vi "PS-RA01B FPGA.vi"() -> ()   [LabVIEW 2011]
uses:
  <vilib>/rvi/eio/common/nirviEmuTemplateMethod_errors.vi
  <vilib>/eio/EIONode/EIONode.xnode
  <vilib>/rvi/Analysis/measure/butterworth/XNode/niFpgaButterworthFilter.xnode
  <vilib>/eio/EIOMethodNode/EIOMethodNode.xnode
panel:
  out "Mod5/AI2":fxp<+/-,20,5> format="%.17g"
  out "Mod5/AI0":fxp<+/-,20,5> format="%.17g"
  out "Mod5/AI1":fxp<+/-,20,5> format="%.17g"
  out "Mod1/AI2":fxp<+/-,20,5> format="%.17g"
  out "Mod1/AI3":fxp<+/-,20,5> format="%.17g"
  out "Mod1/AI0":fxp<+/-,20,5> format="%.17g"
  out "Mod1/AI1":fxp<+/-,20,5> format="%.17g"
  out "Mod5/AI3":fxp<+/-,20,5> format="%.17g"
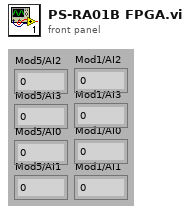
[diagram p1: front panel]
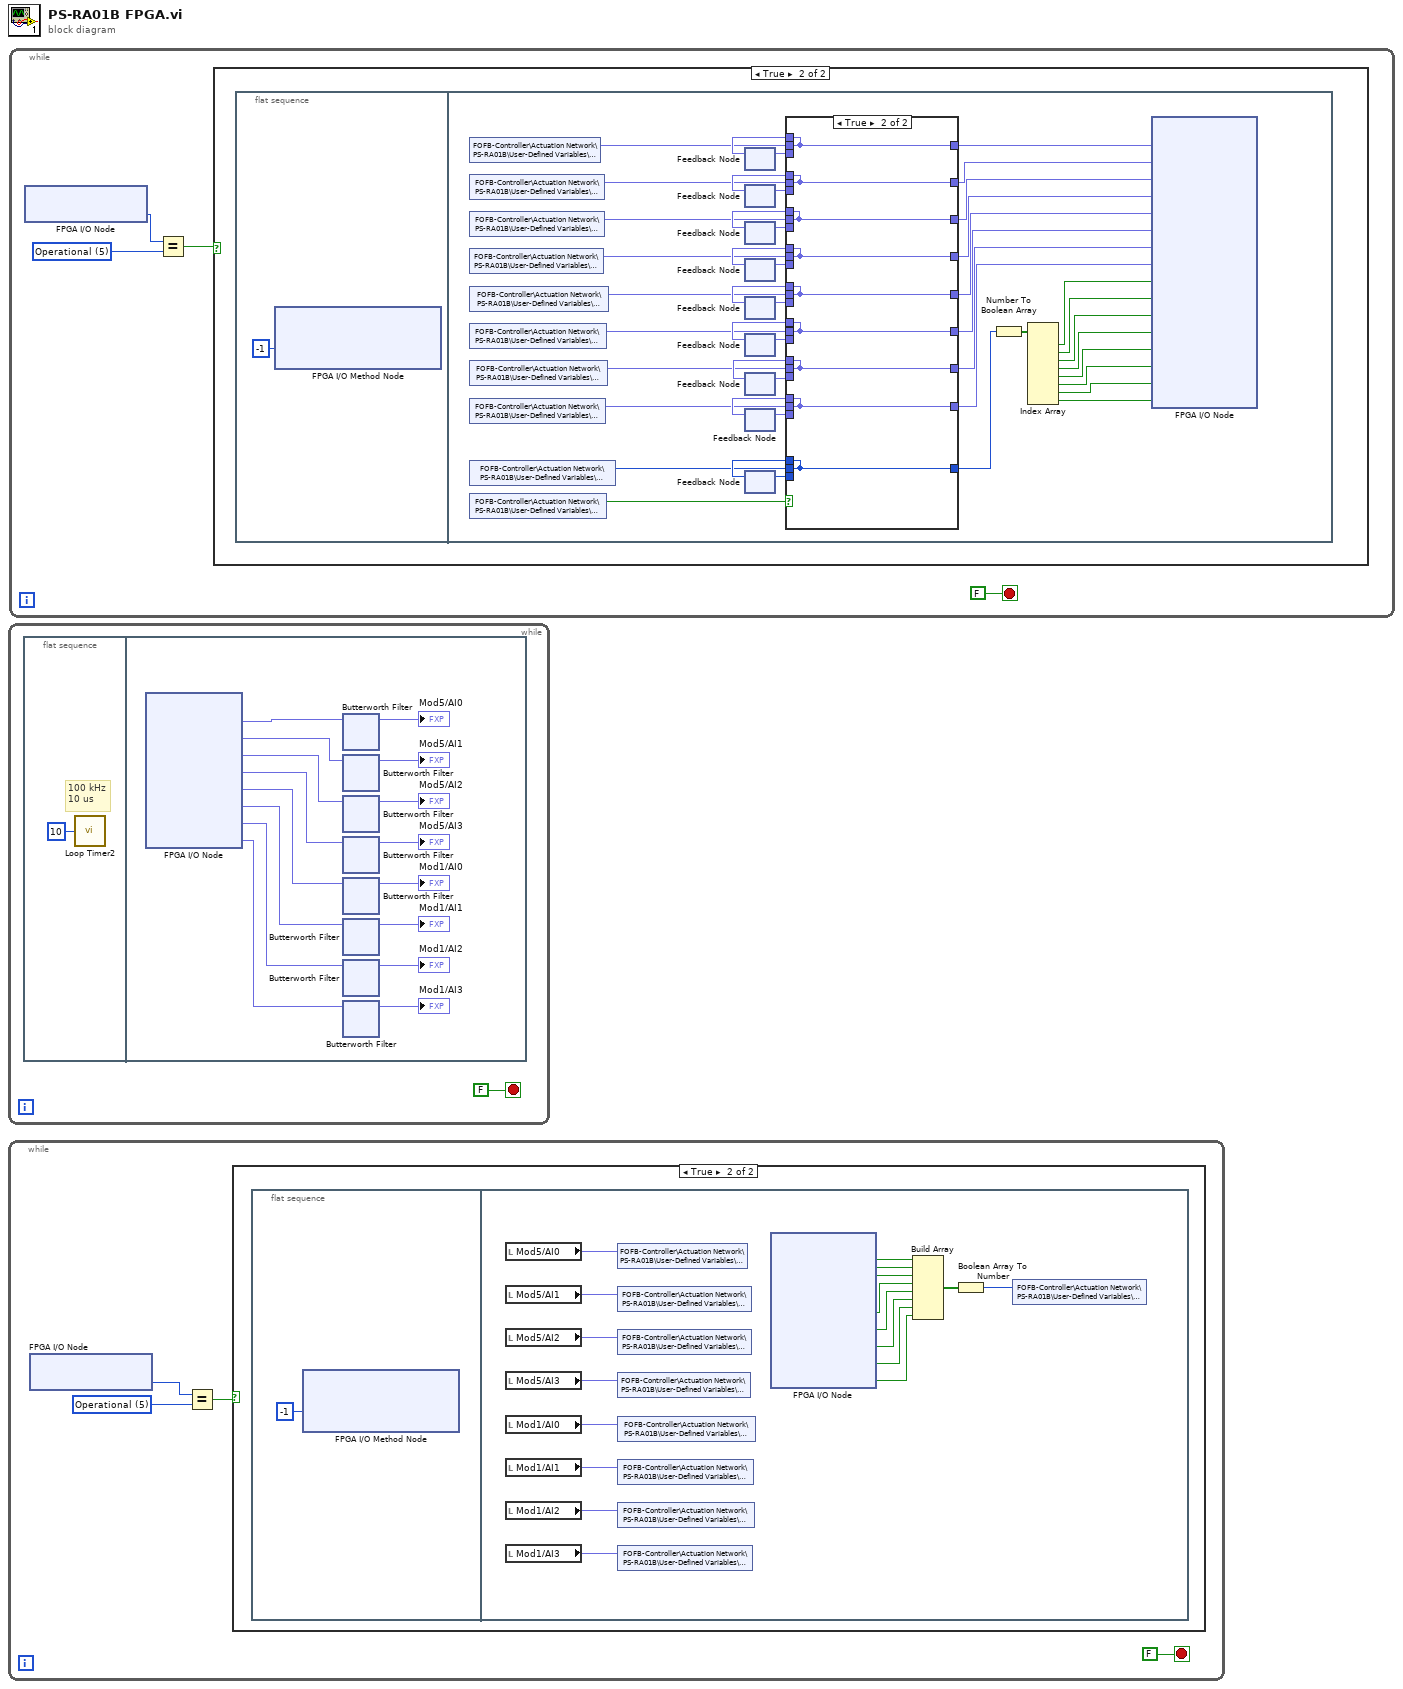
[diagram p0: block diagram]
diagram:
  n1 = while {
    stop <- FALSE stop-if-true
    n2 = flat-sequence {
      frame #0 {
        # "100 kHz\n10 us"
        n3 = call "Loop Timer2"("Count(uSec)"=u8 10) -> ()  [unwired: 1 out]
      }
      frame #1 {
        n4 = xnode "FPGA I/O Node"() -> ("Mod5/AI0"=w18:fxp<+/-,20,5>, "Mod5/AI1"=w17:fxp<+/-,20,5>, "Mod5/AI2"=w16:fxp<+/-,20,5>, "Mod5/AI3"=w15:fxp<+/-,20,5>, "Mod1/AI0"=w14:fxp<+/-,20,5>, "Mod1/AI1"=w13:fxp<+/-,20,5>, "Mod1/AI2"=w12:fxp<+/-,20,5>, "Mod1/AI3"=w11:fxp<+/-,20,5>)  [unwired: 8 in, 8 out]
        n5 = xnode "Butterworth Filter"("input data"=w18) -> ("output data"=→"Mod5/AI0":fxp<+/-,20,5>)  [unwired: 2 in]
        n6 = xnode "Butterworth Filter"("input data"=w17) -> ("output data"=→"Mod5/AI1":fxp<+/-,20,5>)  [unwired: 2 in]
        n7 = xnode "Butterworth Filter"("input data"=w16) -> ("output data"=→"Mod5/AI2":fxp<+/-,20,5>)  [unwired: 2 in]
        n8 = xnode "Butterworth Filter"("input data"=w15) -> ("output data"=→"Mod5/AI3":fxp<+/-,20,5>)  [unwired: 2 in]
        n9 = xnode "Butterworth Filter"("input data"=w14) -> ("output data"=→"Mod1/AI0":fxp<+/-,20,5>)  [unwired: 2 in]
        n10 = xnode "Butterworth Filter"("input data"=w13) -> ("output data"=→"Mod1/AI1":fxp<+/-,20,5>)  [unwired: 2 in]
        n11 = xnode "Butterworth Filter"("input data"=w12) -> ("output data"=→"Mod1/AI2":fxp<+/-,20,5>)  [unwired: 2 in]
        n12 = xnode "Butterworth Filter"("input data"=w11) -> ("output data"=→"Mod1/AI3":fxp<+/-,20,5>)  [unwired: 2 in]
      }
    }
  }
  n13 = while {
    stop <- FALSE stop-if-true
    w77 = u8 5 items=["Init"=1, "PreOp"=2, "Bootstrap"=3, "SafeOp"=4, "Operational"=5]
    n14 = xnode "FPGA I/O Node"() -> ("EtherCAT State"=w76:u8)  [unwired: 1 in, 1 out]
    n15 = Equal?(x=w76, y=w77) -> (x = y?=w75:bool)
    n16 = case shown="True" w75 {
      frame False {
      }
      frame True {
        n17 = flat-sequence {
          frame #0 {
            n18 = xnode "FPGA I/O Method Node"("Timeout"=-1) -> ()  [unwired: 1 in, 2 out]
          }
          frame #1 {
            n19 = local read "Mod5/AI0"() -> (w95:fxp<+/-,20,5>)
            n20 = local read "Mod5/AI1"() -> (w94:fxp<+/-,20,5>)
            n21 = local read "Mod5/AI2"() -> (w93:fxp<+/-,20,5>)
            n22 = local read "Mod5/AI3"() -> (w91:fxp<+/-,20,5>)
            n23 = local read "Mod1/AI0"() -> (w90:fxp<+/-,20,5>)
            n24 = local read "Mod1/AI1"() -> (w89:fxp<+/-,20,5>)
            n25 = local read "Mod1/AI2"() -> (w88:fxp<+/-,20,5>)
            n26 = local read "Mod1/AI3"() -> (w92:fxp<+/-,20,5>)
            n27 = shared-variable "FOFB-Controller\\Actuation Network\\PS-RA01B\\User-Defined Variables\\ACH02-Reading"(w95) -> ()  [unwired: 1 in, 1 out]
            n28 = shared-variable "FOFB-Controller\\Actuation Network\\PS-RA01B\\User-Defined Variables\\RRA01B-Reading"(w94) -> ()  [unwired: 1 in, 1 out]
            n29 = shared-variable "FOFB-Controller\\Actuation Network\\PS-RA01B\\User-Defined Variables\\ALV02A-Reading"(w93) -> ()  [unwired: 1 in, 1 out]
            n30 = shared-variable "FOFB-Controller\\Actuation Network\\PS-RA01B\\User-Defined Variables\\ALV02B-Reading"(w91) -> ()  [unwired: 1 in, 1 out]
            n31 = shared-variable "FOFB-Controller\\Actuation Network\\PS-RA01B\\User-Defined Variables\\ACH03A-Reading"(w90) -> ()  [unwired: 1 in, 1 out]
            n32 = shared-variable "FOFB-Controller\\Actuation Network\\PS-RA01B\\User-Defined Variables\\ACV03A-Reading"(w89) -> ()  [unwired: 1 in, 1 out]
            n33 = shared-variable "FOFB-Controller\\Actuation Network\\PS-RA01B\\User-Defined Variables\\ACH01B-Reading"(w88) -> ()  [unwired: 1 in, 1 out]
            n34 = shared-variable "FOFB-Controller\\Actuation Network\\PS-RA01B\\User-Defined Variables\\ACV01B-Reading"(w92) -> ()  [unwired: 1 in, 1 out]
            n35 = xnode "FPGA I/O Node"() -> ("Mod3/DIO6"=w87:bool, "Mod3/DIO7"=w86:bool, "Mod3/DIO4"=w85:bool, "Mod3/DIO5"=w84:bool, "Mod3/DIO2"=w83:bool, "Mod3/DIO3"=w82:bool, "Mod3/DIO0"=w81:bool, "Mod3/DIO1"=w80:bool)  [unwired: 8 in, 8 out]
            n36 = Build Array(w87, w86, w85, w84, w83, w82, w81, w80) -> (w97:bool[])
            n37 = Boolean Array To Number(Boolean array=w97) -> (number=w96:u8)
            n38 = shared-variable "FOFB-Controller\\Actuation Network\\PS-RA01B\\User-Defined Variables\\PS-RA01B-Status"(w96) -> ()  [unwired: 1 in, 1 out]
          }
        }
      }
    }
  }
  n39 = while {
    stop <- FALSE stop-if-true
    w98 = u8 5 items=["Init"=1, "PreOp"=2, "Bootstrap"=3, "SafeOp"=4, "Operational"=5]
    n40 = xnode "FPGA I/O Node"() -> ("EtherCAT State"=w99:u8)  [unwired: 1 in, 1 out]
    n41 = Equal?(x=w99, y=w98) -> (x = y?=w100:bool)
    n42 = case shown="True" w100 {
      frame False {
      }
      frame True {
        n43 = flat-sequence {
          frame #0 {
            n44 = xnode "FPGA I/O Method Node"("Timeout"=-1) -> ()  [unwired: 1 in, 2 out]
          }
          frame #1 {
            n45 = shared-variable "FOFB-Controller\\Actuation Network\\PS-RA01B\\User-Defined Variables\\ACH02-Setpoint"() -> (w112:fxp<+/-,20,5>)  [unwired: 1 in, 1 out]
            n46 = shared-variable "FOFB-Controller\\Actuation Network\\PS-RA01B\\User-Defined Variables\\RRA01B-Setpoint"() -> (w111:fxp<+/-,20,5>)  [unwired: 1 in, 1 out]
            n47 = shared-variable "FOFB-Controller\\Actuation Network\\PS-RA01B\\User-Defined Variables\\ALV02A-Setpoint"() -> (w110:fxp<+/-,20,5>)  [unwired: 1 in, 1 out]
            n48 = shared-variable "FOFB-Controller\\Actuation Network\\PS-RA01B\\User-Defined Variables\\ALV02B-Setpoint"() -> (w109:fxp<+/-,20,5>)  [unwired: 1 in, 1 out]
            n49 = shared-variable "FOFB-Controller\\Actuation Network\\PS-RA01B\\User-Defined Variables\\ACH03A-Setpoint"() -> (w108:fxp<+/-,20,5>)  [unwired: 1 in, 1 out]
            n50 = shared-variable "FOFB-Controller\\Actuation Network\\PS-RA01B\\User-Defined Variables\\ACV03A-Setpoint"() -> (w107:fxp<+/-,20,5>)  [unwired: 1 in, 1 out]
            n51 = shared-variable "FOFB-Controller\\Actuation Network\\PS-RA01B\\User-Defined Variables\\ACH01B-Setpoint"() -> (w106:fxp<+/-,20,5>)  [unwired: 1 in, 1 out]
            n52 = shared-variable "FOFB-Controller\\Actuation Network\\PS-RA01B\\User-Defined Variables\\ACV01B-Setpoint"() -> (w105:fxp<+/-,20,5>)  [unwired: 1 in, 1 out]
            n53 = shared-variable "FOFB-Controller\\Actuation Network\\PS-RA01B\\User-Defined Variables\\PS-RA01B-ON-OFF"() -> (w104:u8)  [unwired: 1 in, 1 out]
            n54 = shared-variable "FOFB-Controller\\Actuation Network\\PS-RA01B\\User-Defined Variables\\PS-RA01B-Enable"() -> (w103:bool)  [unwired: 1 in, 1 out]
            n55 = feedback #1() -> (w114:fxp<+/-,20,5>)  [unwired: 1 in]
            n56 = feedback #2() -> (w133:fxp<+/-,20,5>)  [unwired: 1 in]
            n57 = feedback #3() -> (w136:fxp<+/-,20,5>)  [unwired: 1 in]
            n58 = feedback #4() -> (w137:fxp<+/-,20,5>)  [unwired: 1 in]
            n59 = feedback #5() -> (w139:fxp<+/-,20,5>)  [unwired: 1 in]
            n60 = feedback #6() -> (w142:fxp<+/-,20,5>)  [unwired: 1 in]
            n61 = feedback #7() -> (w145:fxp<+/-,20,5>)  [unwired: 1 in]
            n62 = feedback #8() -> (w143:fxp<+/-,20,5>)  [unwired: 1 in]
            n63 = feedback #9() -> (w148:u8)  [unwired: 1 in]
            n64 = case shown="True" w103 {
              tunnel: w112 -> [_ w166]
              tunnel: w114 -> [w157 _]
              tunnel: [w157 w166] -> w116
              tunnel: [w156 w165] -> w117
              tunnel: [w149 w164] -> w118
              tunnel: [w155 w159] -> w119
              tunnel: [w150 w160] -> w120
              tunnel: [w154 w161] -> w121
              tunnel: [w153 w162] -> w122
              tunnel: [w152 w163] -> w131
              tunnel: [w151 w158] -> w113
              tunnel: [w157 w166] -> w132
              tunnel: w111 -> [_ w165]
              tunnel: w105 -> [_ w163]
              tunnel: w133 -> [w156 _]
              tunnel: [w156 w165] -> w134
              tunnel: w110 -> [_ w164]
              tunnel: [w149 w164] -> w135
              tunnel: w136 -> [w149 _]
              tunnel: w109 -> [_ w159]
              tunnel: [w155 w159] -> w138
              tunnel: w137 -> [w155 _]
              tunnel: w108 -> [_ w160]
              tunnel: w139 -> [w150 _]
              tunnel: [w150 w160] -> w140
              tunnel: w107 -> [_ w161]
              tunnel: [w154 w161] -> w141
              tunnel: w142 -> [w154 _]
              tunnel: w143 -> [w152 _]
              tunnel: [w152 w163] -> w144
              tunnel: w145 -> [w153 _]
              tunnel: [w153 w162] -> w146
              tunnel: w106 -> [_ w162]
              tunnel: [w151 w158] -> w147
              tunnel: w104 -> [_ w158]
              tunnel: w148 -> [w151 _]
              frame False {
              }
              frame True {
              }
            }
            n65 = feedback-in #1(w132) -> ()
            n66 = feedback-in #2(w134) -> ()
            n67 = feedback-in #3(w135) -> ()
            n68 = feedback-in #4(w138) -> ()
            n69 = feedback-in #5(w140) -> ()
            n70 = feedback-in #6(w141) -> ()
            n71 = feedback-in #7(w146) -> ()
            n72 = feedback-in #8(w144) -> ()
            n73 = feedback-in #9(w147) -> ()
            n74 = Number To Boolean Array(number=w113) -> (Boolean array=w115:bool[])
            n75 = Index Array(array=w115) -> (element #1=w123:bool, element #2=w124:bool, element #3=w125:bool, element #4=w126:bool, element #5=w130:bool, element #6=w127:bool, element #7=w128:bool, element #8=w129:bool)  [unwired: 8 in]
            n76 = xnode "FPGA I/O Node"("Mod6/AO0"=w116, "Mod6/AO1"=w117, "Mod6/AO2"=w118, "Mod6/AO3"=w119, "Mod2/AO0"=w120, "Mod2/AO1"=w121, "Mod2/AO2"=w122, "Mod2/AO3"=w131, "Mod4/DIO6"=w123, "Mod4/DIO7"=w124, "Mod4/DIO4"=w125, "Mod4/DIO5"=w126, "Mod4/DIO2"=w130, "Mod4/DIO3"=w127, "Mod4/DIO0"=w128, "Mod4/DIO1"=w129) -> ()  [unwired: 16 in, 16 out]
          }
        }
      }
    }
  }
